vi "Send Write to Database.vi"(7 "Message Priority (Normal)":T2=enum."Normal", 8 "error in (no error)":errorcluster, 10 "DB to Write":T1[](array[typedef]), 11 "Message Enqueuer":refnum<class "Message Enqueuer.lvclass">) -> (0 "error out":errorcluster, 3 "Message Enqueuer out":refnum<class "Message Enqueuer.lvclass">)   [LabVIEW 2023, in "Central Data Manager.lvlib" / "Write to Database Msg.lvclass"]
doc: "This VI sends the message to an actor."
uses:
  Write to Database Msg.lvclass
  <vilib>/ActorFramework/Message Enqueuer/Message Enqueuer.lvclass
  <vilib>/ActorFramework/Message Enqueuer/Message Priority.ctl
  File Data Manager/File Data Manager/Database Selection.ctl
  C:/Program Files/National Instruments/LabVIEW 2023/vi.lib/ActorFramework/Message/Message.lvclass
  Write to Database Msg.lvclass/Write to Database Msg.ctl
  <vilib>/ActorFramework/Message Enqueuer/Message Enqueuer.lvclass/Message Enqueuer.ctl
  <vilib>/ActorFramework/Message Priority Queue/Priority Enqueue.vi
  C:/Users/bhaghyaraj/Trainings/NI Actor Framework/SDLC/Central Data Manager/Central Data Manager Messages/Write to Database Msg/Write to Database Msg.lvclass
  Central Data Manager/Central Data Manager.lvclass
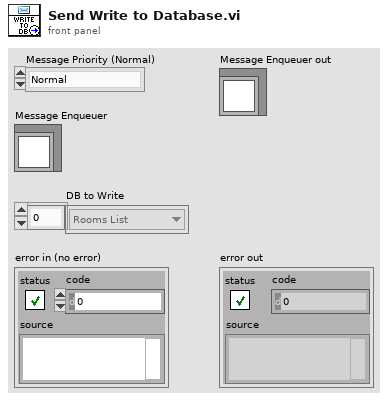
[diagram p1: front panel]
types:
  T1 = typedef "Central Data Manager.lvlib/Central Data Manager.lvclass/Database Selection.ctl" = enum16{"Rooms List", "Guests History"}
  T2 = typedef "Actor Framework.lvlib/Message Enqueuer.lvclass/Message Priority.ctl" = enum16{"Low", "Normal", "High"}
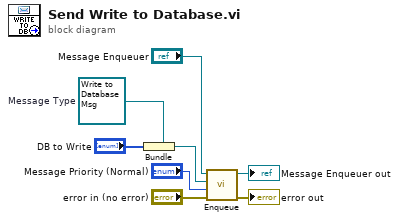
[diagram p0: block diagram]
diagram:
  w5 = refnum<class "Write to Database Msg.lvclass"> refnum  # Message Type
  n1 = Bundle(cluster=w5, "DB to Write") -> (w4:refnum<class "Write to Database Msg.lvclass">)
  n2 = call <vilib>:"Enqueue.vi"("error in (no error)"="error in (no error)", "Message Priority (Normal)"="Message Priority (Normal)", "Message"=w4, "Message Enqueuer in"="Message Enqueuer") -> ("error out"=→"error out":errorcluster, "Message Enqueuer in"=→"Message Enqueuer out":refnum<class "Message Enqueuer.lvclass">)  [unwired: 6 in]
